vi "FileIO-Change dB SL to dB HL.vi"(0 "selected path in":path, 11 "error in (no error)":errorcluster) -> (4 "selected path out":path, 15 "error out":errorcluster)   [LabVIEW 2020]
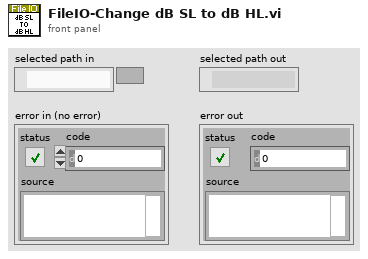
[diagram p1: front panel]
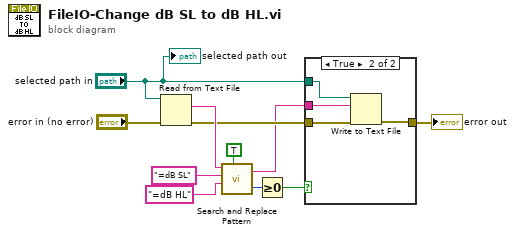
[diagram p0: block diagram]
diagram:
  n1 = Read from Text File(file (use dialog)="selected path in", error in="error in (no error)") -> (text=w10:string, error out=w4:errorcluster)  [unwired: 2 in, 2 out]
  n2 = call <vilib>:"Search and Replace Pattern.vi"("string"=w10, "regular expression (\"\")"="=dB SL" ("regular expression (\"\")"), "replace string (\"\")"="=dB HL" ("replace string (\"\")"), "replace all? (F)"=TRUE) -> ("result string"=w1:string, "offset past match"=w6:i32)  [unwired: 1 in]
  n3 = Greater Or Equal To 0?(x=w6) -> (x >= 0?=w5:bool)
  n4 = case shown="True" w5 {
    tunnel: "selected path in" -> [_ w15]
    tunnel: w4 -> [w12 w16]
    tunnel: [w12 w14] -> w3
    tunnel: w1 -> [_ w13]
    frame False {
    }
    frame True {
      n5 = Write to Text File(file (use dialog)=w15, text=w13, error in=w16) -> (error out=w14:errorcluster)  [unwired: 1 in, 2 out]
    }
  }
  "error out" <- w3
  "selected path out" <- "selected path in"
